vi "RecordPointsJoyStick.vi"() -> ()   [LabVIEW 2019]
uses:
  Other Models/2010/Motion/AbortSingle.vi
panel:
  out "Positions":string
  in  "Finish":bool
  in  "StopJoyStick":bool
  out "String":string
  out "error out":errorcluster
  in  "OutputFile":path=path "C:/Users/TTUHEP/Documents/LabVIEW/GantryPrograms/Configs/temp.txt"
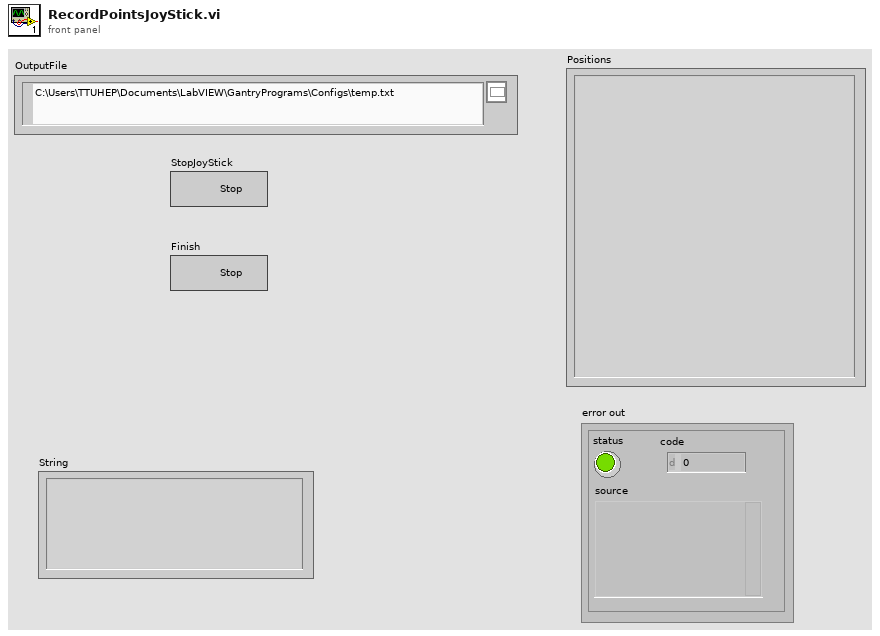
[diagram p1: front panel]
types:
  T1 = enum16{"open", "replace", "create", "open or create", "replace or create", "replace or create with confirmation"}
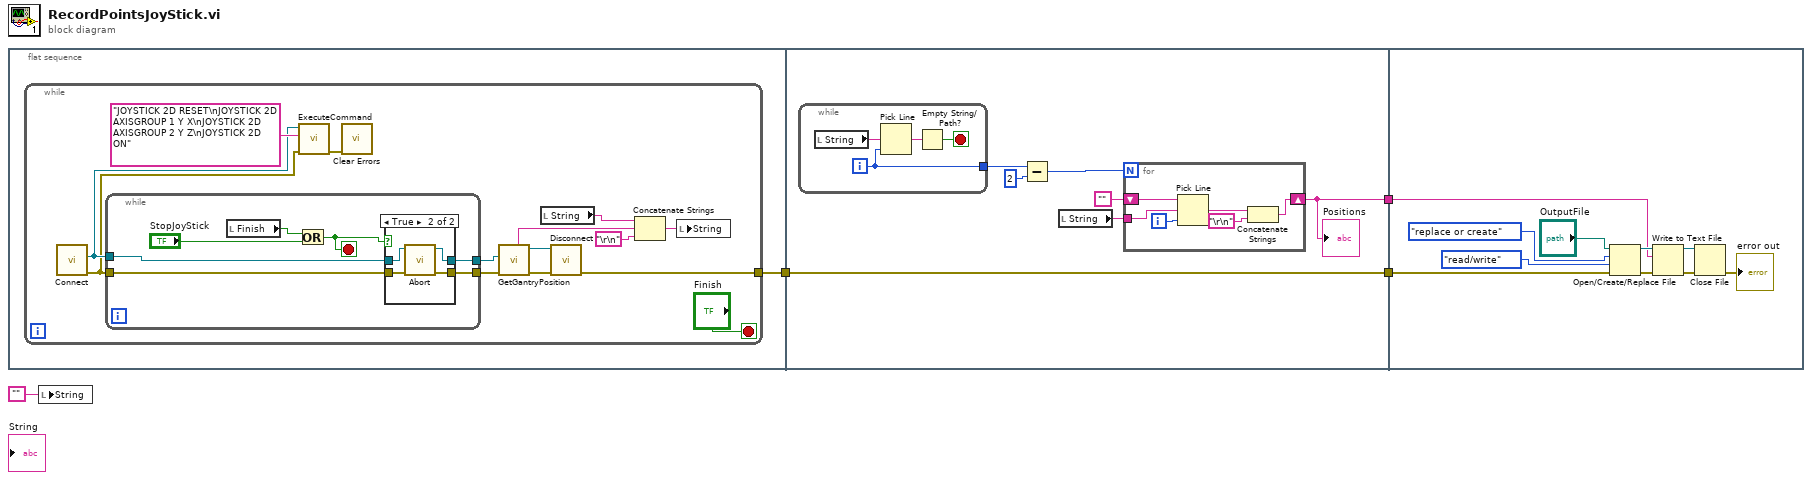
[diagram p0: block diagram]
diagram:
  n1 = flat-sequence {
    tunnel: [w5] -> w3
    tunnel: w3 -> [w34]
    tunnel: [w34] -> w2
    tunnel: [w33] -> w1
    tunnel: w2 -> [w52]
    tunnel: w1 -> [w50]
    frame #0 {
      n2 = while {
        tunnel: [w10] -> w5
        stop <- "Finish" stop-if-true
        n3 = call "Connect.vi"() -> ("error out"=w16:errorcluster, "controller"=w17:refnum<k24>)  [unwired: 10 in]
        n4 = while {
          tunnel: w17 -> [w26]
          tunnel: [w25] -> w14
          tunnel: [w24] -> w15
          tunnel: w16 -> [w23]
          stop <- w22 stop-if-true
          n5 = local read "Finish"() -> (w20:bool)
          n6 = Or(x=w20, y="StopJoyStick") -> (x .or. y?=w22:bool)
          n7 = case shown="True" w22 {
            tunnel: w26 -> [w28 w32]
            tunnel: w23 -> [w27 w31]
            tunnel: [w27 w30] -> w25
            tunnel: [w28 w29] -> w24
            frame False {
            }
            frame True {
              n8 = call-poly "Abort.vi"("error in (no error)"=w31, "controller in"=w32) -> ("error out"=w30:errorcluster, "controller out"=w29:refnum<k24>)  [unwired: 8 in]
            }
          }
        }
        n9 = call "ExecuteCommand.vi"("error in (no error)"=w16, "Command Code"="JOYSTICK 2D RESET\nJOYSTICK 2D AXISGROUP 1 Y X\nJOYSTICK 2D AXISGROUP 2 Y Z\nJOYSTICK 2D ON", "controller in"=w17) -> ("error out"=w18:errorcluster)  [unwired: 6 in, 2 out]
        n10 = call <vilib>:"Clear Errors.vi"("error in (no error)"=w18) -> ()  [unwired: 5 in, 2 out]
        n11 = call "GetGantryPosition.vi"("error in (no error)"=w14, "Controller In"=w15) -> ("error out"=w13:errorcluster, "controller out"=w12:refnum<k24>, "Position_XYZ"=w11:string)  [unwired: 3 in, 4 out]
        n12 = local read "String"() -> (w8:string)
        n13 = call "Disconnect.vi"("error in (no error)"=w13, "controller"=w12) -> ("error out"=w10:errorcluster)  [unwired: 9 in]
        n14 = Concatenate Strings(w8, w11, "\r\n") -> (w6:string)
        n15 = local write "String"(w6) -> ()
      }
    }
    frame #1 {
      n16 = while {
        tunnel: [w46] -> w39
        i -> [w46]
        stop <- w47 stop-if-true
        n17 = local read "String"() -> (w49:string)
        n18 = Pick Line(multi-line string=w49, line index=w46) -> (output string=w48:string)  [unwired: 1 in]
        n19 = Empty String/Path?(string/path=w48) -> (empty?=w47:bool)
      }
      n20 = Subtract(x=w39, y=2) -> (x-y=w37:i32)
      n21 = local read "String"() -> (w36:string)
      n22 = for {
        N: w37 -> [_]
        tunnel: w36 -> [w44]
        shift-right: [w40] -> w33
        shift-left: "" -> [w43]
        i -> [w45]
        n23 = Pick Line(string ("")=w43, multi-line string=w44, line index=w45) -> (output string=w42:string)
        n24 = Concatenate Strings(w42, "\r\n") -> (w40:string)
      }
      "Positions" <- w33
    }
    frame #2 {
      n25 = Open/Create/Replace File(file path (use dialog)="OutputFile", error in=w52, operation (0:open)=T1."replace or create", access (0:read/write)=enum16{"read/write", "read-only", "write-only"}."read/write") -> (refnum out=w56:refnum<file>, error out=w57:errorcluster)  [unwired: 2 in, 1 out]
      n26 = Write to Text File(file (use dialog)=w56, text=w50, error in=w57) -> (refnum out=w59:refnum<file>, error out=w58:errorcluster)  [unwired: 1 in, 1 out]
      n27 = Close File(refnum=w59, error in=w58) -> (error out=→"error out":errorcluster)  [unwired: 1 out]
    }
  }
  n28 = local write "String"("") -> ()
